vi "Ask Price.vi"(8 "error in (no error)":errorcluster, 11 "Customer A in":refnum<class "Customer A.lvclass">) -> (0 "error out":errorcluster, 3 "Customer A out":refnum<class "Customer A.lvclass">)   [LabVIEW 2020, in "Customer A.lvlib" / "Customer A.lvclass"]
uses:
  Customer A.lvclass
  Customer A.lvclass/Customer A.ctl
  <vilib>/ActorFramework/Message Enqueuer/Message Enqueuer.lvclass/Message Enqueuer.ctl
  <vilib>/ActorFramework/Message Enqueuer/Enqueue.vi
  ShopAssistant/ShopAssistant Messages/ShopAssistantAnswer Msg/ShopAssistantAnswer Msg.lvclass
  E:/Program Files (x86)/National Instruments/LabVIEW 2020/vi.lib/ActorFramework/Message/Message.lvclass
  <vilib>/ActorFramework/Message Priority Queue/Priority Enqueue.vi
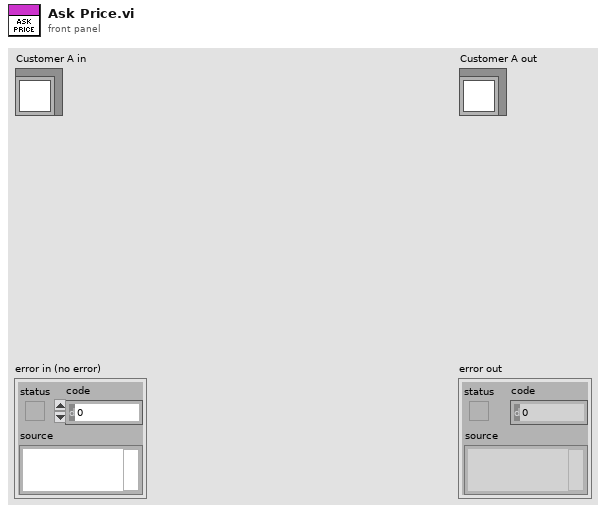
[diagram p1: front panel]
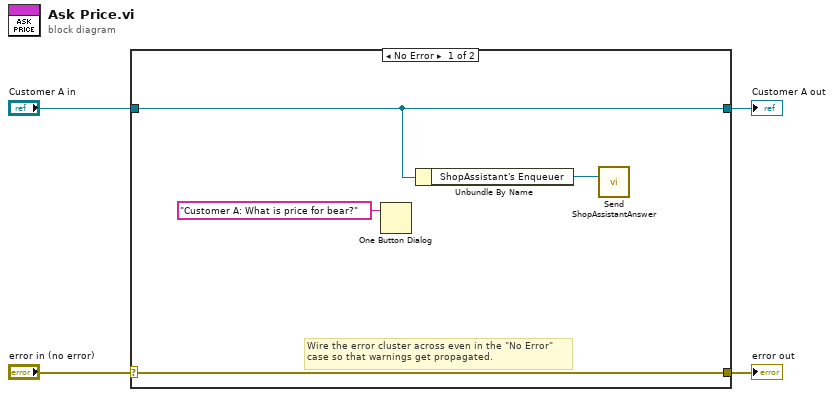
[diagram p0: block diagram]
diagram:
  n1 = case shown="No Error" "error in (no error)" {
    selector: "error in (no error)" -> [w8 w10]
    tunnel: [w8 w10] -> w3
    tunnel: [w6 w9] -> w1
    tunnel: "Customer A in" -> [w6 w9]
    frame No Error {
      # "Wire the error cluster across even in the \"No Error\"\ncase so that warnings get propagated."
      n2 = One Button Dialog(message="Customer A: What is price for bear?") -> ()  [unwired: 1 in, 1 out]
      n3 = Unbundle By Name(w6) -> ("ShopAssistant's Enqueuer"=w5:refnum<class "Message Enqueuer.lvclass">)
      n4 = call "Send ShopAssistantAnswer.vi"("Message Enqueuer"=w5) -> ()  [unwired: 9 in, 2 out]
    }
    frame Error {
    }
  }
  "error out" <- w3
  "Customer A out" <- w1
